vi "Globals.vi"() -> ()   [LabVIEW 2024, in "Sift Stream.lvlib" / "Sift Stream.lvclass"]
uses:
  Sift Stream.lvclass
panel:
  in  "Sample Rate":string
  in  "Sift API Key":string
  in  "Sift API URL":string
  in  "Asset Name":string
  in  "Select channels":string="Select channels"
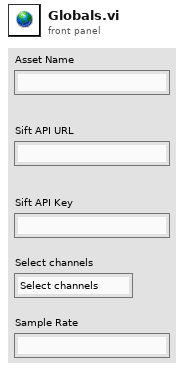
[diagram p1: front panel]
diagram:
